vi "Feed_Intake_Brain.vi"(8 "Station_Pickup":bool, 9 "Ele_At_Pos":bool, 10 "Tote_Detect_2":bool, 11 "Tote_Detect_1":bool) -> (0 "Open_Infeed":bool, 1 "Infeed_cmd":dbl, 2 "Pickup_2_Auto":bool, 3 "Station_Auto":bool)   [LabVIEW 2014]
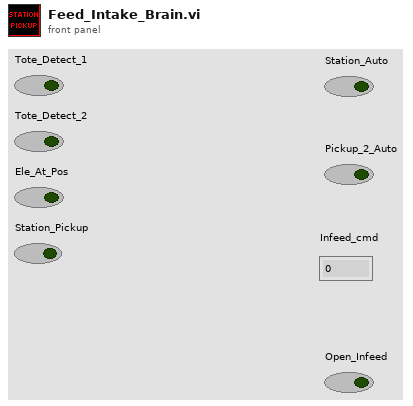
[diagram p1: front panel]
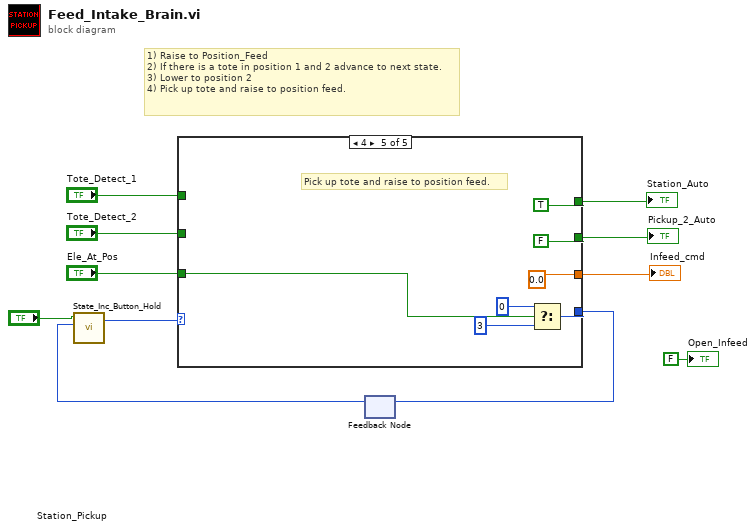
[diagram p0: block diagram]
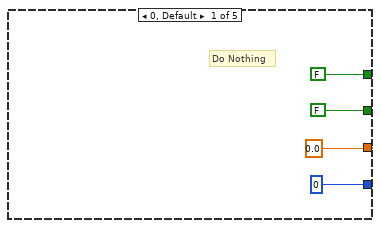
[diagram p2: hidden frame]
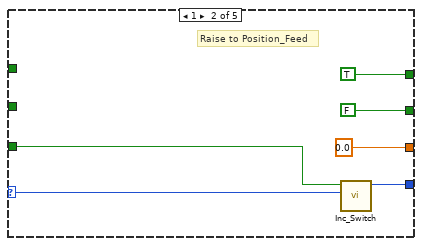
[diagram p3: hidden frame]
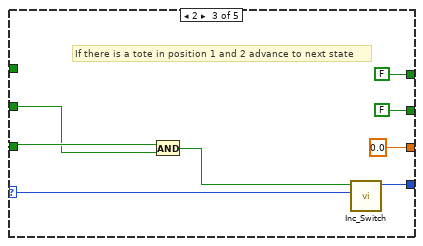
[diagram p4: hidden frame]
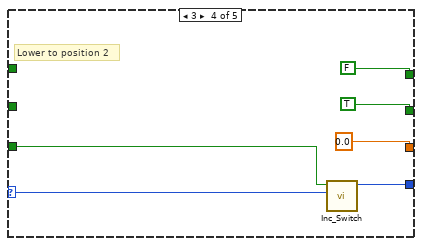
[diagram p5: hidden frame]
diagram:
  # "1) Raise to Position_Feed\n2) If there is a tote in position 1 and 2 advance to next state.\n3) Lower to position 2\n4) Pick up tote and raise to position feed."
  n1 = feedback #1() -> (w2:i32)  [unwired: 1 in]
  n2 = call "State_Inc_Button_Hold.vi"("Numeric in"=w2, "Floor_Pickup"="Station_Pickup") -> ("t"=w4:i32)  [unwired: 9 in]
  n3 = case shown="4" w4 {
    selector: w4 -> [_ w17 w23 w30 _]
    tunnel: [FALSE TRUE FALSE FALSE TRUE] -> w11
    tunnel: "Ele_At_Pos" -> [_ w18 _ w32 w42]
    tunnel: [0 w16 w22 w31 w41] -> w7
    tunnel: [FALSE FALSE FALSE TRUE FALSE] -> w9
    tunnel: [0.0 0.0 0.0 0.0 0.0] -> w8
    tunnel: "Tote_Detect_1" -> [_ _ w27 _ _]
    tunnel: "Tote_Detect_2" -> [_ _ w26 _ _]
    frame 0, Default {
      # "Do Nothing"
    }
    frame 1 {
      # "Raise to Position_Feed"
      n4 = call "Inc_Switch.vi"("Numeric in"=w17, "Ele_At_Pos"=w18) -> ("Numeric out"=w16:i32)  [unwired: 9 in]
    }
    frame 2 {
      # "If there is a tote in position 1 and 2 advance to next state"
      n5 = And(x=w27, y=w26) -> (x .and. y?=w24:bool)
      n6 = call "Inc_Switch.vi"("Numeric in"=w23, "Ele_At_Pos"=w24) -> ("Numeric out"=w22:i32)  [unwired: 9 in]
    }
    frame 3 {
      # "Lower to position 2"
      n7 = call "Inc_Switch.vi"("Numeric in"=w30, "Ele_At_Pos"=w32) -> ("Numeric out"=w31:i32)  [unwired: 9 in]
    }
    frame 4 {
      # "Pick up tote and raise to position feed."
      n8 = Select(t=0, s=w42, f=3 ("t")) -> (s? t:f=w41:i32)
    }
  }
  "Station_Auto" <- w11
  "Pickup_2_Auto" <- w9
  "Infeed_cmd" <- w8
  n9 = feedback-in #1(w7) -> ()
  "Open_Infeed" <- FALSE ("Open_Infeed")
